vi "Close.vi"(8 "error in (no error)":errorcluster, 11 "Teledyne-T3AFG120 in":refnum<class "Teledyne-T3AFG120.lvclass">) -> (0 "error out":errorcluster, 3 "Teledyne-T3AFG120 out":refnum<class "Teledyne-T3AFG120.lvclass">)   [LabVIEW 2023, in "Teledyne-T3AFG120.lvlib" / "Teledyne-T3AFG120.lvclass"]
uses:
  Teledyne-T3AFG120.lvclass
  Teledyne-T3AFG120.lvclass/Teledyne-T3AFG120.ctl
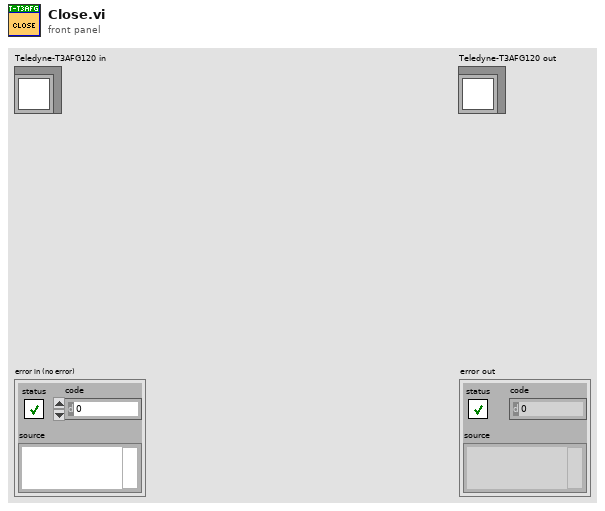
[diagram p1: front panel]
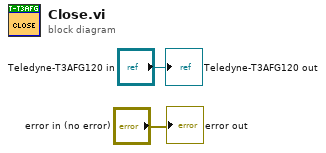
[diagram p0: block diagram]
diagram:
  "error out" <- "error in (no error)"
  "Teledyne-T3AFG120 out" <- "Teledyne-T3AFG120 in"
